vi "Teleop.vi"(10 "Match Info":T1={"Autonomous Elapsed Seconds"=0.0, "TeleOp Elapsed Seconds"=0.0, "Disabled Elapsed Seconds"=0.0, "Visited Autonomous"=FALSE, "Visited TeleOp"=FALSE, "Visited Disabled"=FALSE, "Autonomous Settings"={"Autonomous Style"=enum."Independent", "VI Refnum"=refnum}}, 11 "Call Context":T2) -> ()   [LabVIEW 2014]
doc: "This VI is called for each TeleOp packet received from the DS where the robot is not disabled. It is often used to read from the joysticks and update I/O or to update setpoints for timed control loops. It should complete and return within 20 milliseconds or it may miss DS packets."
uses:
  <vilib>/Rock Robotics/WPI/DriverStation/WPI_DriverStationDerivedRobotMode.ctl
  <vilib>/Rock Robotics/WPI/DriverStation/WPI_DriverStationMatch Info.ctl
  Robot Global Data.vi
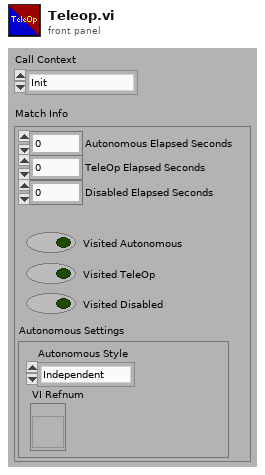
[diagram p1: front panel]
types:
  T1 = typedef "WPI_DriverStationMatch Info.ctl" = cluster{"Autonomous Elapsed Seconds":dbl, "TeleOp Elapsed Seconds":dbl, "Disabled Elapsed Seconds":dbl, "Visited Autonomous":bool, "Visited TeleOp":bool, "Visited Disabled":bool, "Autonomous Settings":cluster{"Autonomous Style":enum16{"Iterative", "Independent"}, "VI Refnum":refnum<vi>}}
  T2 = typedef "WPI_DriverStationDerivedRobotMode.ctl" = enum16{"Init", "Execute", "Stop"}
  T3 = cluster{"axis 3 (throttle)":dbl, "axis 1 (x)":dbl, "axis 2 (y)":dbl}
  T4 = cluster{"Trigger":bool, "Top 1":bool, "Side Trigger":bool, "Top 2":bool, "Top 3":bool, "Top 4":bool, "Bottom 1":bool, "Bottom 2":bool, "Bottom 3":bool, "Bottom 4":bool, "Bottom 5":bool, "Bottom 6":bool}
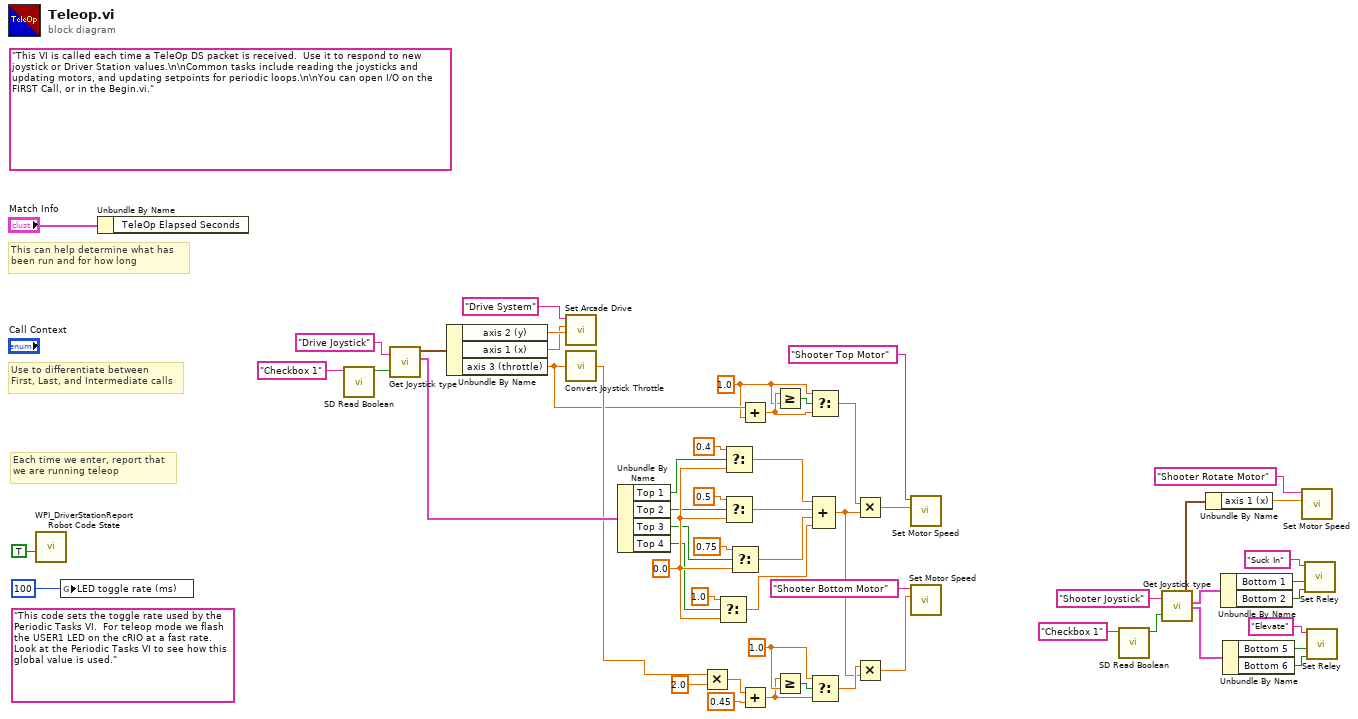
[diagram p0: block diagram]
diagram:
  w31 = 1.0 ("y")
  w1 = 1.0 ("y")
  w47 = 0.0 ("t")
  (unwired) "This code sets the toggle rate used by the Periodic Tasks VI.  For teleop mode we flash the USER1 LED on the cRIO at a fast rate.  Look at the Periodic Tasks VI to see how this global value is used."
  (unwired) "This VI is called each time a TeleOp DS packet is received.  Use it to respond to new joystick or Driver Station values.\n\nCommon tasks include reading the joysticks and updating motors, and updating setpoints for periodic loops.\n\nYou can open I/O on the FIRST Call, or in the Begin.vi."
  # "Each time we enter, report that\nwe are running teleop"
  # "Use to differentiate between\nFirst, Last, and Intermediate calls"
  # "This can help determine what has\nbeen run and for how long"
  n1 = call <vilib>:"WPI_DriverStationReport Robot Code State.vi"("TeleOp"=TRUE ("Autonomous")) -> ()  [unwired: 10 in, 1 out]
  n2 = global write "Robot Global Data.vi" "LED toggle rate (ms)"(u32 100 ("LED ms toggle rate")) -> ()
  n3 = Unbundle By Name("Match Info") -> ()  [unwired: 1 out]
  n4 = call <vilib>:"SD Read Boolean.vi"("Name"="Checkbox 1" ("refnum name")) -> ("Boolean"=w50:bool)  [unwired: 8 in, 2 out]
  n5 = call "Get Joystick type.vi"("refnum name"="Drive Joystick", "Pro Joystick"=w50) -> ("Axes"=w48:T3, "Buttons"=w49:T4)  [unwired: 2 in]
  n6 = Unbundle By Name(w48) -> ("axis 2 (y)"=w17:dbl, "axis 1 (x)"=w16:dbl, "axis 3 (throttle)"=w36:dbl)
  n7 = call "Set Arcade Drive.vi"("Y axis value"=w17, "X axis value"=w16, "refnum name"="Drive System") -> ()  [unwired: 9 in]
  n8 = call "Convert Joystick Throttle.vi"("Input"=w36) -> ("Output"=w37:dbl)
  n9 = Unbundle By Name(w49) -> ("Top 1"=w46:bool, "Top 2"=w45:bool, "Top 3"=w44:bool, "Top 4"=w43:bool)
  n10 = Multiply(x=w37, y=2.0) -> (x*y=w26:dbl)
  n11 = Select(t=1.0, s=w43, f=w47) -> (s? t:f=w5:dbl)
  n12 = Select(t=0.4, s=w46, f=w47) -> (s? t:f=w2:dbl)
  n13 = Select(t=0.5, s=w45, f=w47) -> (s? t:f=w3:dbl)
  n14 = Select(t=0.75, s=w44, f=w47) -> (s? t:f=w4:dbl)
  n15 = Add(x=w36, y=w1) -> (x+y=w34:dbl)
  n16 = Add(x=w26, y=0.45) -> (x+y=w25:dbl)
  n17 = Greater Or Equal?(x=w34, y=w1) -> (x >= y?=w35:bool)
  n18 = Greater Or Equal?(x=w25, y=w31) -> (x >= y?=w32:bool)
  n19 = Select(t=w1, s=w35, f=w34) -> (s? t:f=w33:dbl)
  n20 = Select(t=w31, s=w32, f=w25) -> (s? t:f=w30:dbl)
  n21 = Compound Arithmetic op=ADD(w2, w3, w4, w5) -> (w6:dbl)
  n22 = Multiply(x=w33, y=w6) -> (x*y=w23:dbl)
  n23 = Multiply(x=w30, y=w6) -> (x*y=w19:dbl)
  n24 = call "Set Motor Speed.vi"("Output"=w23, "refnum name"="Shooter Top Motor") -> ()  [unwired: 10 in]
  n25 = call "Set Motor Speed.vi"("Output"=w19, "refnum name"="Shooter Bottom Motor") -> ()  [unwired: 10 in]
  n26 = call <vilib>:"SD Read Boolean.vi"("Name"="Checkbox 1" ("refnum name")) -> ("Boolean"=w27:bool)  [unwired: 8 in, 2 out]
  n27 = call "Get Joystick type.vi"("refnum name"="Shooter Joystick", "Pro Joystick"=w27) -> ("Axes"=w7:T3, "Buttons"=w11:T4)  [unwired: 2 in]
  n28 = Unbundle By Name(w7) -> ("axis 1 (x)"=w21:dbl)
  n29 = Unbundle By Name(w11) -> ("Bottom 1"=w13:bool, "Bottom 2"=w14:bool)
  n30 = Unbundle By Name(w11) -> ("Bottom 5"=w9:bool, "Bottom 6"=w10:bool)
  n31 = call "Set Motor Speed.vi"("Output"=w21, "refnum name"="Shooter Rotate Motor") -> ()  [unwired: 10 in]
  n32 = call "Set Reley.vi"("Reverse"=w14, "Forward"=w13, "refnum name"="Suck In") -> ()  [unwired: 9 in]
  n33 = call "Set Reley.vi"("Reverse"=w10, "Forward"=w9, "refnum name"="Elevate") -> ()  [unwired: 9 in]
